vi "VI ref template for message processing.vi"(8 "message data":variant, 10 "message":string, 11 "message type":string) -> ()   [LabVIEW 2016, in "Message Queue.lvlib"]
uses:
  Message Queue.lvlib
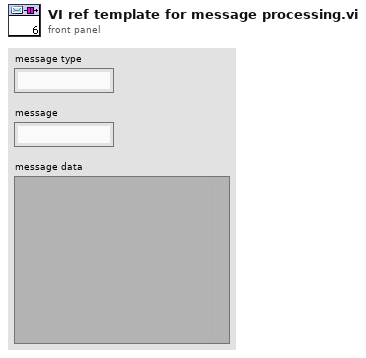
[diagram p1: front panel]
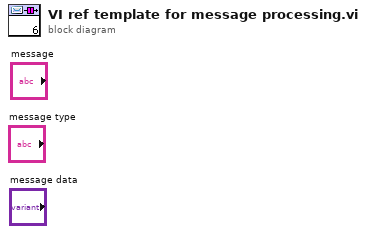
[diagram p0: block diagram]
diagram:
